vi "Start Command.vi"(8 "error in (no error)":errorcluster, 11 "Drive by Power in":refnum<class "Drive by Power.lvclass">) -> (0 "error out":errorcluster, 3 "Drive by Power out":refnum<class "Drive by Power.lvclass">)   [LabVIEW 2013, in "Logical Systems.lvlib" / "Drive Train.lvlib" / "Drive by Power.lvlib" / "Drive by Power.lvclass"]
uses:
  Drive by Power.lvclass
  Drive Train Command/Drive Train Command Class/Drive Train Command.lvclass
  Drive by Power.lvclass/Drive by Power.ctl
  Drive Train Messages/Set Power Msg/Set Power Msg.lvclass/Set Power Msg.ctl
  <vilib>/ActorFramework/Message Enqueuer/Message Enqueuer.lvclass/Message Enqueuer.ctl
  <vilib>/ActorFramework/Actor/Actor.lvclass/Actor.ctl
  <vilib>/ActorFramework/Message Enqueuer/Enqueue.vi
  <vilib>/ActorFramework/Message Enqueuer/Init from Existing Queue.vi
  <vilib>/ActorFramework/Message Priority Queue/Priority Enqueue.vi
  Drive Train Messages/Set Power Msg/Set Power Msg.lvclass
  <vilib>/ActorFramework/Message Enqueuer/Message Enqueuer.lvclass
  Robot Actors/Command/Command Messages/Finish Command Msg/Finish Command Msg.lvclass
  <vilib>/ActorFramework/Actor/Actor.lvclass
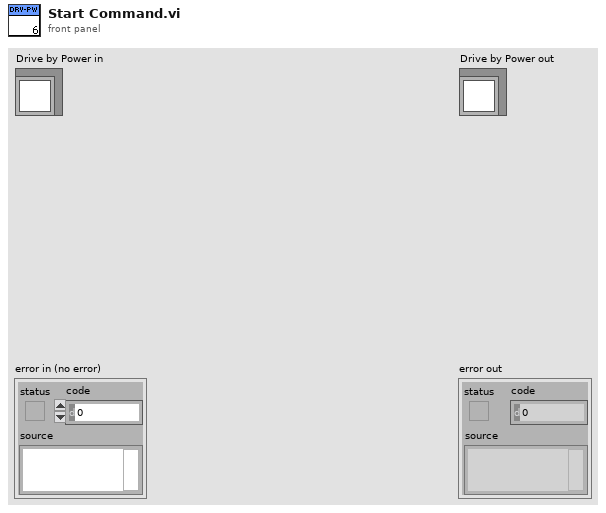
[diagram p1: front panel]
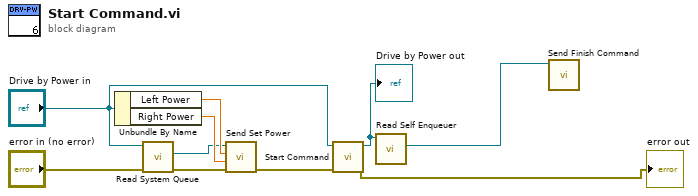
[diagram p0: block diagram]
diagram:
  n1 = Unbundle By Name("Drive by Power in") -> ("Left Power"=w10:dbl, "Right Power"=w9:dbl)
  n2 = call-dynamic "Read System Queue.vi"("error in (no error)"="error in (no error)", "Command in"="Drive by Power in") -> ("error out"=w6:errorcluster, "Actor Framework:Message Enqueuer"=w8:refnum<class "Message Enqueuer.lvclass">)  [unwired: 7 in, 1 out]
  n3 = call "Send Set Power.vi"("error in (no error)"=w6, "Right Power"=w9, "Left Power"=w10, "Message Enqueuer"=w8) -> ("error out"=w3:errorcluster)  [unwired: 6 in, 1 out]
  n4 = call-parent "Start Command.vi"("error in (no error)"=w3, "Command in"="Drive by Power in") -> ("error out"=→"error out":errorcluster, "Command out"=w4:refnum<class "Drive by Power.lvclass">)  [unwired: 8 in]
  "Drive by Power out" <- w4
  n5 = call <vilib>:"Read Self Enqueuer.vi"("Actor"=w4) -> ("Self Enqueuer"=w1:refnum<class "Message Enqueuer.lvclass">)  [unwired: 10 in]
  n6 = call "Send Finish Command.vi"("Message Enqueuer"=w1) -> ()  [unwired: 9 in, 2 out]
